vi "buffer 2D array clust.vi"(0 "Array":i32[][](array[numeric]), 1 "History length":i32, 2 "Log":T1=enum."TimeStamp", 10 "Start channel":i32) -> ()   [LabVIEW 2018]
uses:
  history_array_type.ctl
  CAEN globals.vi
panel:
  out "Numeric":i32
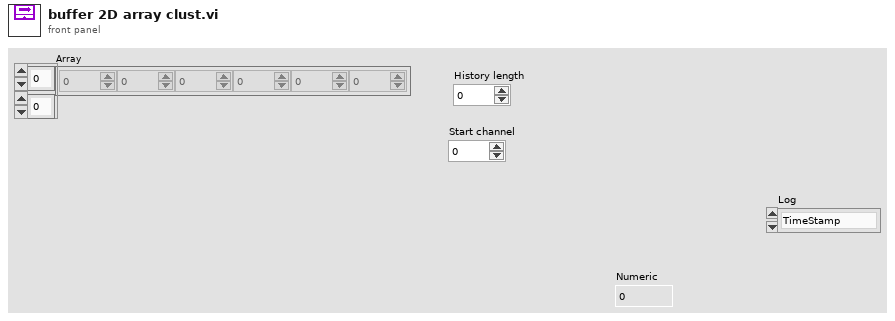
[diagram p1: front panel]
types:
  T1 = typedef "history_array_type.ctl" = enum16{"Vmon", "Vset", "Imon", "Iset", "TimeStamp"}
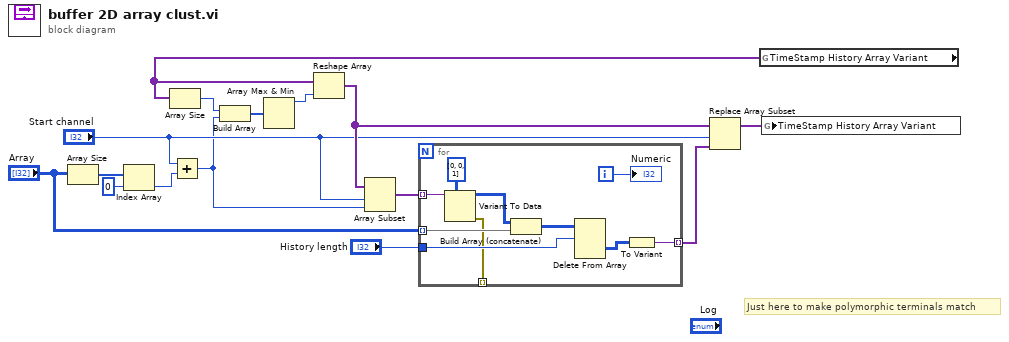
[diagram p0: block diagram]
diagram:
  # "Just here to make polymorphic terminals match"
  n1 = Array Size(array="Array") -> (size(s)=w7:i32[])
  n2 = Index Array(array=w7, index=0) -> (element=w6:i32)
  n3 = Add(x="Start channel", y=w6) -> (x+y=w4:i32)
  n4 = global read "CAEN globals.vi" "TimeStamp History Array Variant"() -> (w1:variant[])
  n5 = Array Size(array=w1) -> (size(s)=w13:i32)
  n6 = Build Array(w13, w4) -> (w14:i32[])
  n7 = Array Max & Min(array=w14) -> (max value=w15:i32)  [unwired: 3 out]
  n8 = Reshape Array(w1, w15) -> (w12:variant[])
  n9 = Array Subset(array=w12, index="Start channel", length=w4) -> (w3:variant[])
  n10 = for {
    tunnel: w3 -> [w25] mode=indexing
    tunnel: "Array" -> [w23] mode=indexing
    tunnel: [w21] -> w11 mode=indexing
    tunnel: "History length" -> [w19]
    tunnel: [w16] -> _ mode=indexing
    i -> [w17]
    n11 = Variant To Data(type=i32[][] [[0, 0, 1]] ("Value"), Variant=w25) -> (data=w22:i32[][], error out=w16:errorcluster)  [unwired: 1 in]
    n12 = Build Array (concatenate)(w22, w23) -> (w20:i32[][])
    n13 = Delete From Array(array=w20, length=w19) -> (deleted portion=w18:i32[][])  [unwired: 2 in, 1 out]
    n14 = To Variant(anything=w18) -> (Variant=w21:variant)
    "Numeric" <- w17
  }
  n15 = Replace Array Subset(array=w12, new element=w11, index="Start channel") -> (w2:variant[])
  n16 = global write "CAEN globals.vi" "TimeStamp History Array Variant"(w2) -> ()
